vi "UTIL_Timebase.vi"(10 "Reset":bool, 11 "Sample Rate":dbl) -> (3 "Time(ms)":dbl)   [LabVIEW 2024]
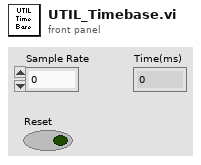
[diagram p1: front panel]
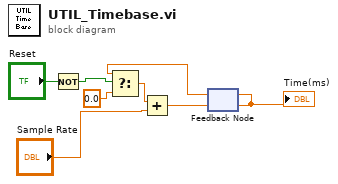
[diagram p0: block diagram]
diagram:
  n1 = Not(x="Reset") -> (.not. x?=w2:bool)
  n2 = feedback #1() -> (w4:dbl)  [unwired: 1 in]
  n3 = Select(t=w4, s=w2, f=0.0) -> (s? t:f=w5:dbl)
  n4 = Add(x=w5, y="Sample Rate") -> (x+y=w7:dbl)
  "Time(ms)" <- w7
  n5 = feedback-in #1(w7) -> ()
